vi "Begin.vi"(8 "error in":errorcluster) -> (0 "error out":errorcluster)   [LabVIEW 2017]
doc: "Called before other user functions, this VI can be used to open I/O refnums, load in file data, and do general program initialization. Notice that the <B>error out</B> terminal is simply used for data flow. Wiring it to other structures or subVIs ensures that this VI runs first."
uses:
  <vilib>/Rock Robotics/WPI/DriverStation/WPI_DriverStationRobotMode2.ctl
  <vilib>/Rock Robotics/WPI/Joystick/WPI_JoystickDeviceEnum.ctl
  <vilib>/Rock Robotics/SystemInterfaces/DIO/FPGA_DIOChannel.ctl
  Robot Global Data.vi
  <vilib>/Rock Robotics/Network Tables/NT Write String Array.vi
  <vilib>/Rock Robotics/WPI/Switch/WPI_SwitchOpenLimit.vi
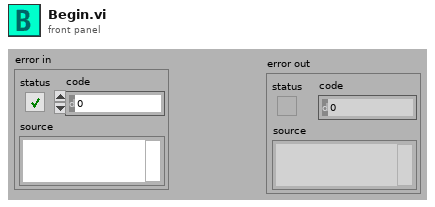
[diagram p1: front panel]
types:
  T1 = typedef "FPGA_DIOChannel.ctl" = enum8{"DIO 0", "DIO 1", "DIO 2", "DIO 3", "DIO 4", "DIO 5", "DIO 6", "DIO 7", "DIO 8", "DIO 9", "DIO MXP 0", "DIO MXP 1", "DIO MXP 2", "DIO MXP 3", "DIO MXP 4", "DIO MXP 5", "DIO MXP 6", "DIO MXP 7", "DIO MXP 8", "DIO MXP 9", "DIO MXP 10", "DIO MXP 11", "DIO MXP 12", "DIO MXP 13", "DIO MXP 14", "DIO MXP 15", "SPI Port CS1", "SPI Port CS2", "SPI Port CS3", "SPI Port MISO", "SPI Port MOSI", "Invalid"}
  T2 = typedef "WPI_JoystickDeviceEnum.ctl" = enum16{"USB 0", "USB 1", "USB 2", "USB 3", "USB 4", "USB 5"}
  T3 = typedef "WPI_DriverStationRobotMode2.ctl" = enum16{"Autonomous Disabled", "Autonomous Enabled", "Teleop Disabled", "Teleop Enabled", "Disconnected", "Finish", "Test Disabled", "Test Enabled", "Emergency Stopped"}
  T4 = typedef "WPI_JoystickDevRef.ctl" = cluster{"Device":T2}
  T5 = typedef "WPI_SwitchDevRef.ctl" = cluster{"DevStatus":errorcluster, "DIO Channel":T1, "CntIndex":T6, "Normally Closed":bool}
  T6 = typedef "FPGA_CounterCtrSystemIndex.ctl" = enum8{"Ctr 0", "Ctr 1", "Ctr 2", "Ctr 3", "Ctr 4", "Ctr 5", "Ctr 6", "Ctr 7", "Invalid"}
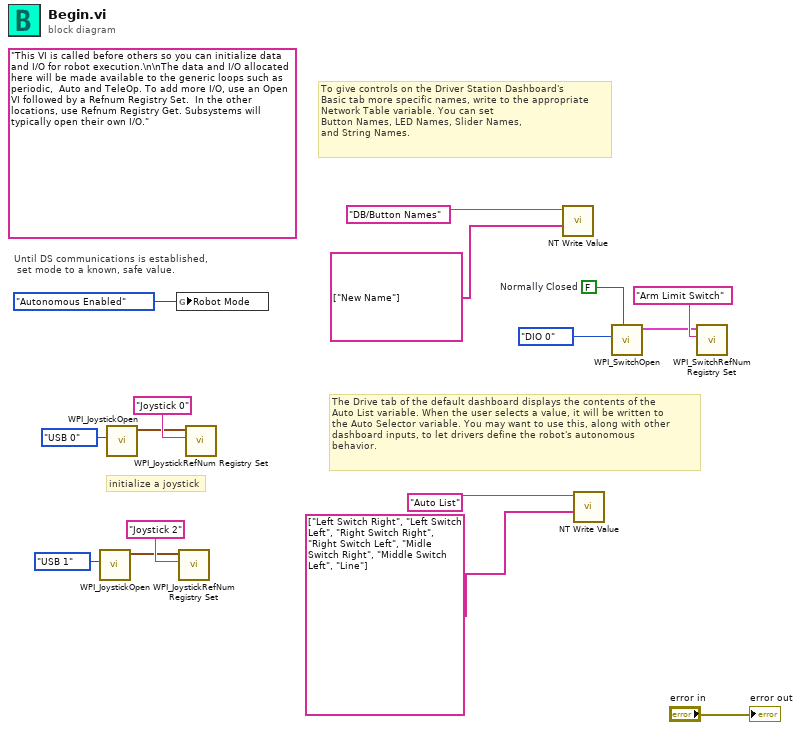
[diagram p0: block diagram]
diagram:
  w2 = FALSE  # Normally Closed
  (unwired) "This VI is called before others so you can initialize data and I/O for robot execution.\n\nThe data and I/O allocated here will be made available to the generic loops such as periodic,  Auto and TeleOp. To add more I/O, use an Open VI followed by a Refnum Registry Set.  In the other locations, use Refnum Registry Get. Subsystems will typically open their own I/O."
  # "The Drive tab of the default dashboard displays the contents of the\nAuto List variable. When the user selects a value, it will be written to\nthe Auto Selector variable. You may want to use this, along with other\ndashboard inputs, to let drivers define the robot's autonomous\nbehavior."
  # "To give controls on the Driver Station Dashboard's\nBasic tab more specific names, write to the appropriate\nNetwork Table variable. You can set\nButton Names, LED Names, Slider Names,\nand String Names."
  # "initialize a joystick"
  # "Until DS communications is established,\n set mode to a known, safe value."
  n1 = call <vilib>:"WPI_JoystickOpen.vi"("JoystickDevice"=WPI_JoystickDeviceEnum."USB 1") -> ("JoystickDevRef"=w6:T4)  [unwired: 10 in]
  n2 = call <vilib>:"WPI_JoystickOpen.vi"("JoystickDevice"=WPI_JoystickDeviceEnum."USB 0") -> ("JoystickDevRef"=w14:T4)  [unwired: 10 in]
  n3 = global write "Robot Global Data.vi" "Robot Mode"(WPI_DriverStationRobotMode2."Autonomous Enabled" ("Robot Mode")) -> ()
  n4 = call <vilib>:"WPI_JoystickRefNum Registry Set.vi"("refnum name"="Joystick 2", "JoystickDevRef"=w6) -> ()  [unwired: 8 in, 2 out]
  n5 = call <vilib>:"WPI_JoystickRefNum Registry Set.vi"("refnum name"="Joystick 0", "JoystickDevRef"=w14) -> ()  [unwired: 8 in, 2 out]
  n6 = call-poly <vilib>:"NT Write Value.vi"("String Array"=string[] ["New Name"], "Name"="DB/Button Names") -> ()  [unwired: 9 in, 1 out]
  n7 = call-poly <vilib>:"NT Write Value.vi"("String Array"=string[] ["Left Switch Right", "Left Switch Left", "Right Switch Right", "Right Switch Left", "Midle Switch Right", "Middle Switch Left", "Line"], "Name"="Auto List") -> ()  [unwired: 9 in, 1 out]
  n8 = call-poly <vilib>:"WPI_SwitchOpen.vi"("Normally Closed"=w2, "DIO Channel"=FPGA_DIOChannel."DIO 0") -> ("SwitchDevRef"=w3:T5)  [unwired: 8 in, 1 out]
  n9 = call <vilib>:"WPI_SwitchRefNum Registry Set.vi"("refnum name"="Arm Limit Switch", "SwitchDevRef"=w3) -> ()  [unwired: 8 in, 2 out]
  "error out" <- "error in"
